vi "NML VISA Close.vi"(8 "Error In":errorcluster, 11 "VISA resource name":refnum<visa-resource-name>) -> (0 "Error Out":errorcluster)   [LabVIEW 2023]
uses:
  Sub Controls/VISA Session Status.ctl
  <vilib>/Instr/_visa.llb/VISA GPIB Control REN Mode.ctl
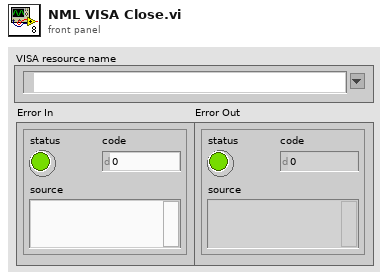
[diagram p1: front panel]
types:
  T1 = typedef "VISA Session Status.ctl" = enum16{"VISA Session Closed", "VISA Session Open", "VISA Session Locked"}
  T2 = typedef "VISA GPIB Control REN Mode.ctl" = u16
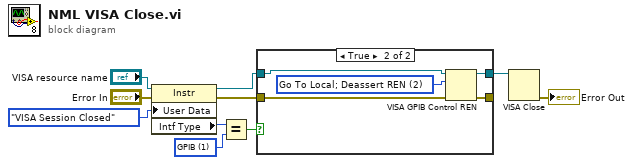
[diagram p0: block diagram]
diagram:
  w3 = u16 1 items=["GPIB"=1, "VXI"=2, "GPIB-VXI"=3, "Serial"=4, "PXI"=5, "TCPIP"=6, "USB"=7, "FireWire"=9] ("Interface Information:Interface Type")
  n1 = property class="Instr"(reference="VISA resource name", error in="Error In", "User Data"=VISA_Session_Status."VISA Session Closed") -> (reference out=w7:refnum<visa-resource-name>, error out=w5:errorcluster, "Intf Type"=w4:u16)
  n2 = Equal?(x=w4, y=w3) -> (x = y?=w2:bool)
  n3 = case shown="True" w2 {
    tunnel: w7 -> [w12 w16]
    tunnel: [w12 w15] -> w6
    tunnel: w5 -> [w11 w14]
    tunnel: [w11 w13] -> _
    frame False {
    }
    frame True {
      w17 = T2 2 items=["Deassert REN", "Assert REN", "Go To Local; Deassert REN ", "Assert REN; Address Device", "Local Lockout (Addressed Devices)", "Local Lockout (This Device)", "Go To Local"] ("Mode")
      n4 = VISA GPIB Control REN(8:w14, 10:w17, 11:w16) -> (0:w13:errorcluster, 3:w15:refnum<visa-resource-name>)
    }
  }
  n5 = VISA Close(VISA resource name=w6) -> (error out=→"Error Out":errorcluster)  [unwired: 1 in]
